vi "CRYListbox Add Item.vi"(9 "Check In":bool[](array[boolean]), 10 "Items In":string[](array[string]), 11 "Candidate item In":string) -> (0 "Cancel operation Out":bool, 1 "Check Out":bool[](array[boolean]), 2 "Items Out":string[](array[string]))   [LabVIEW 2013]
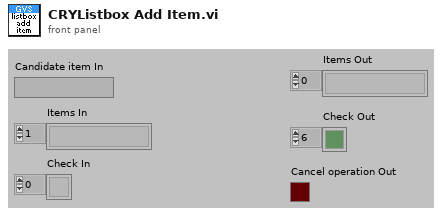
[diagram p1: front panel]
types:
  T1 = enum16{"OK", "Yes", "YesNo", "YesNoCancel", "ReplaceAppend"}
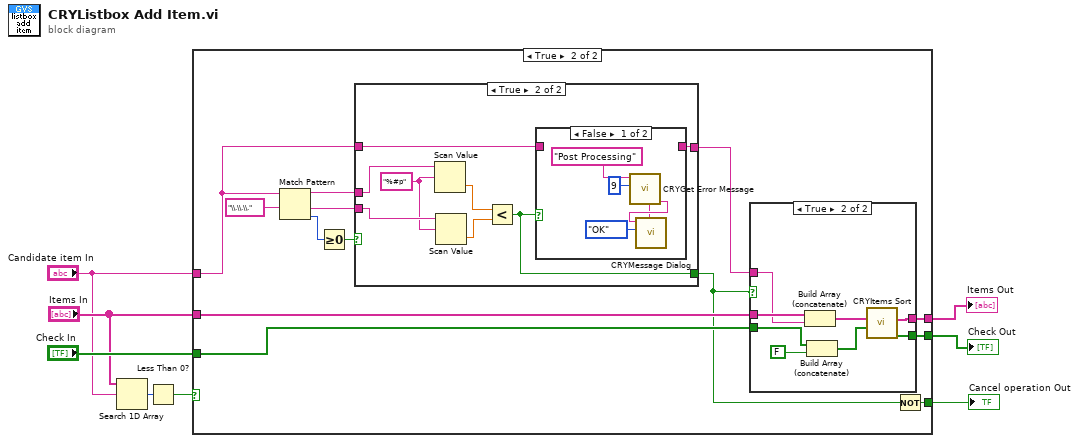
[diagram p0: block diagram]
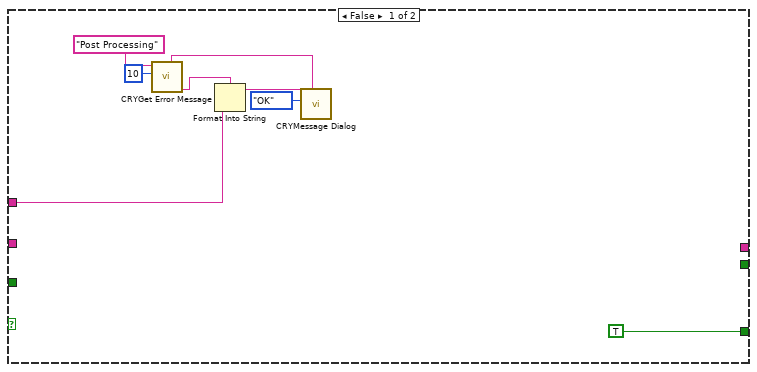
[diagram p2: hidden frame]
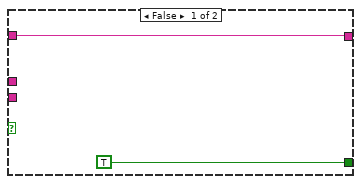
[diagram p4: hidden frame]
diagram:
  n1 = Search 1D Array(1D array="Items In", element="Candidate item In") -> (index of element=w1:i32)  [unwired: 1 in]
  n2 = Less Than 0?(x=w1) -> (x < 0?=w8:bool)
  n3 = case shown="True" w8 {
    tunnel: "Candidate item In" -> [w16 w26]
    tunnel: "Items In" -> [_ w22]
    tunnel: "Check In" -> [_ w21]
    tunnel: [TRUE w25] -> w6
    tunnel: [_ w20] -> w5
    tunnel: [_ w17] -> w4
    frame False {
      n4 = call "CRYGet Error Message.vi"("Error No"=10, "Kind"="Post Processing") -> ("Message Sub 3"=w12:string, "Window Title"=w9:string)  [unwired: 4 in, 4 out]
      n5 = Format Into String(format string=w12, w16) -> (resulting string=w11:string)  [unwired: 2 in, 1 out]
      n6 = call "CRYMessage Dialog.vi"("Window Title"=w9, "YesNoCancel"=T1."OK", "Message Content"=w11) -> ()  [unwired: 7 in, 2 out]
    }
    frame True {
      n7 = Match Pattern(string=w26, regular expression="\\.\\.\\.") -> (before substring=w24:string, after substring=w23:string, offset past match=w28:i32)  [unwired: 2 out]
      n8 = Greater Or Equal To 0?(x=w28) -> (x >= 0?=w27:bool)
      n9 = case shown="True" w27 {
        tunnel: w26 -> [w38 w46]
        tunnel: [TRUE w47] -> w18
        tunnel: w24 -> [_ w44]
        tunnel: w23 -> [_ w43]
        tunnel: [w38 w45] -> w19
        frame False {
        }
        frame True {
          w42 = "%#p" ("format string")
          n10 = Scan Value(string=w44, format string=w42) -> (value=w41:dbl)  [unwired: 1 in, 1 out]
          n11 = Scan Value(string=w43, format string=w42) -> (value=w40:dbl)  [unwired: 1 in, 1 out]
          n12 = Less?(x=w41, y=w40) -> (x < y?=w47:bool)
          n13 = case shown="False" w47 {
            tunnel: w46 -> [_ w53]
            tunnel: [_ w53] -> w45
            frame False {
              n14 = call "CRYGet Error Message.vi"("Error No"=9, "Kind"="Post Processing") -> ("Message Sub 3"=w50:string, "Window Title"=w49:string)  [unwired: 4 in, 4 out]
              n15 = call "CRYMessage Dialog.vi"("Window Title"=w49, "YesNoCancel"=T1."OK", "Message Content"=w50) -> ()  [unwired: 7 in, 2 out]
            }
            frame True {
            }
          }
        }
      }
      n16 = case shown="True" w18 {
        tunnel: w22 -> [_ w37]
        tunnel: [_ w31] -> w20
        tunnel: w21 -> [_ w35]
        tunnel: w19 -> [_ w34]
        tunnel: [_ w30] -> w17
        frame False {
        }
        frame True {
          n17 = Build Array (concatenate)(w37, w34) -> (w33:string[])
          n18 = Build Array (concatenate)(w35, FALSE) -> (w32:bool[])
          n19 = call "CRYItems Sort.vi"("Check In"=w32, "Items In"=w33) -> ("Check Out"=w30:bool[], "Items Out"=w31:string[])  [unwired: 1 in, 7 out]
        }
      }
      n20 = Not(x=w18) -> (.not. x?=w25:bool)
    }
  }
  "Cancel operation Out" <- w6
  "Items Out" <- w5
  "Check Out" <- w4
